vi "OP500InitParam.vi"(8 "errin":errorcluster, 11 "pathin":path) -> (0 "errout":errorcluster caption="error out")   [LabVIEW 2020]
uses:
  VG/VG_ISOmin.vi
  ZEN8 Semi Auto EMC/OP700/VG/VG_TCellmin.vi
  ZEN8 Semi Auto EMC/OP700/VG/VG_TCellmax.vi
  VG/VG_TusineMin.vi
  VG/VG_TusineMax.vi
  VG/VG_VCellMin30.vi
  VG/VG_VCellMax30.vi
  VG/VG_VCellMin70.vi
  VG/VG_VCellMax70.vi
  VG/VG_DeltaTcell.vi
  VG/VG_DeltaVcell.vi
  VG/VG_DCIRmin.vi
  VG/VG_DCIRmax.vi
  VG/VG_OCV30max.vi
  VG/VG_OCV30min.vi
  VG/VG_OCV70max.vi
  VG/VG_OCV70min.vi
  VG/VG_DCIRCurrent.vi
  VG/VG_EquipementsNeeded.vi
  VG/VG_DCIR+OUIouNON.vi
  VG/VG_OP400.vi
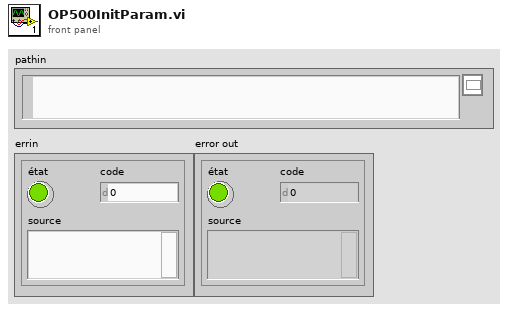
[diagram p1: front panel]
types:
  T1 = cluster{"[0]":dbl, "[1]":dbl, "[2]":dbl, "[3]":dbl, "[4]":dbl, "[5]":dbl, "[6]":dbl, "[7]":dbl, "[8]":dbl}
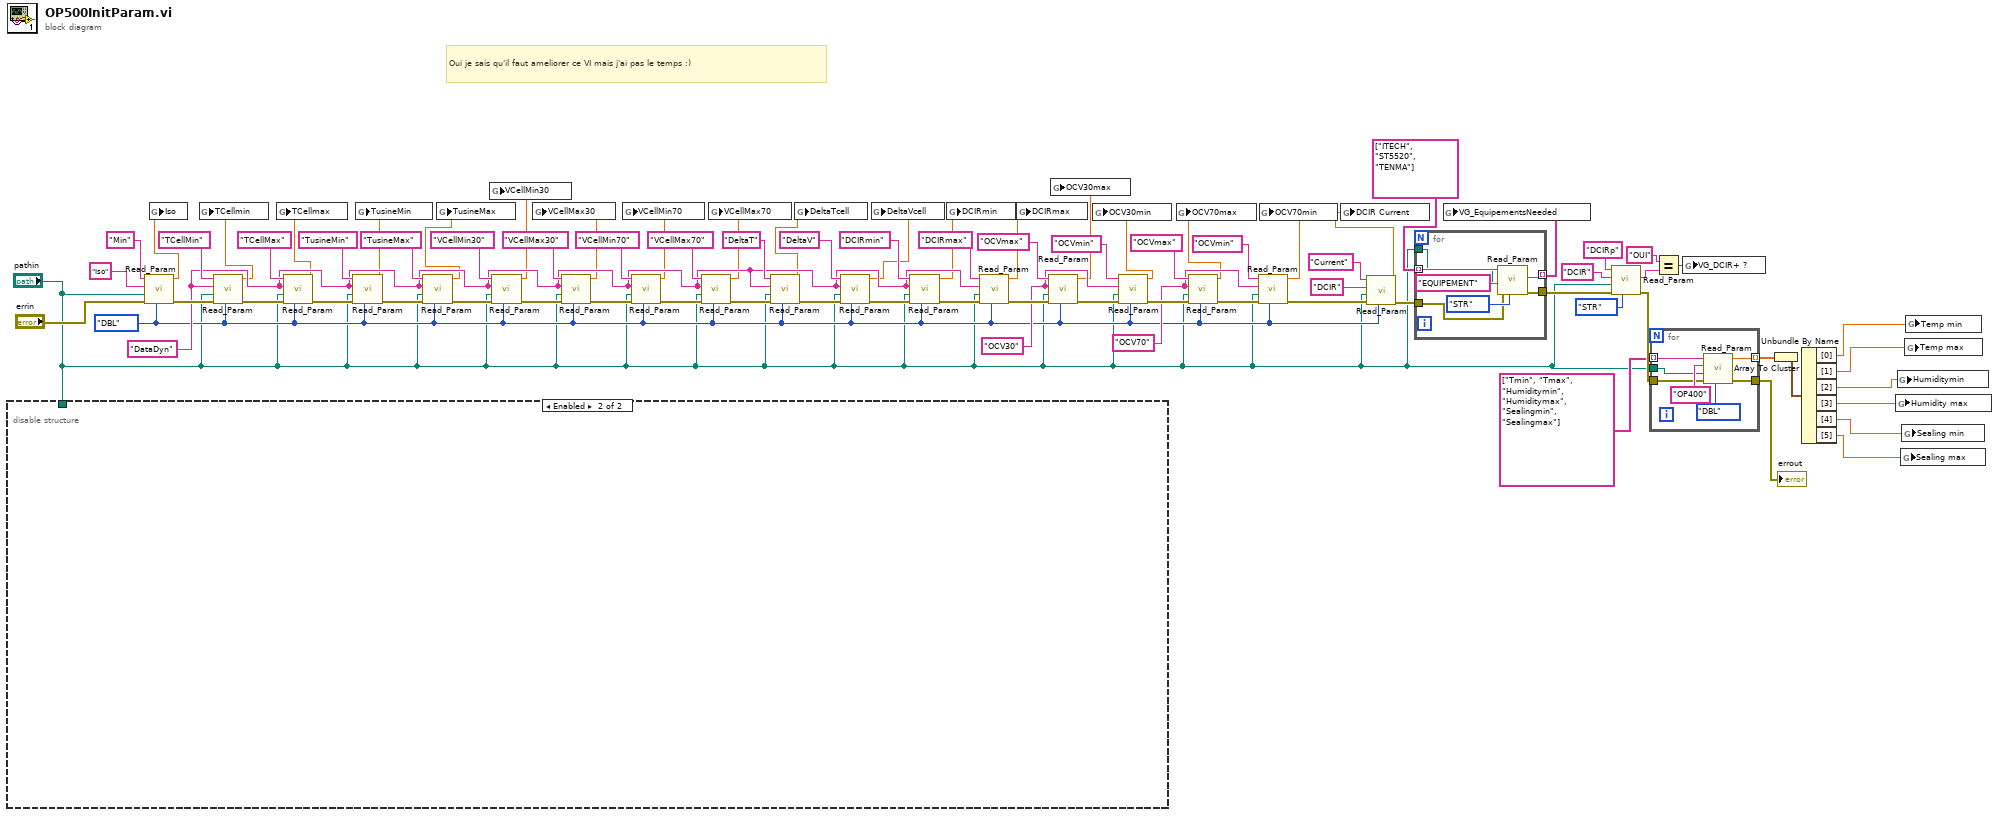
[diagram p0: block diagram]
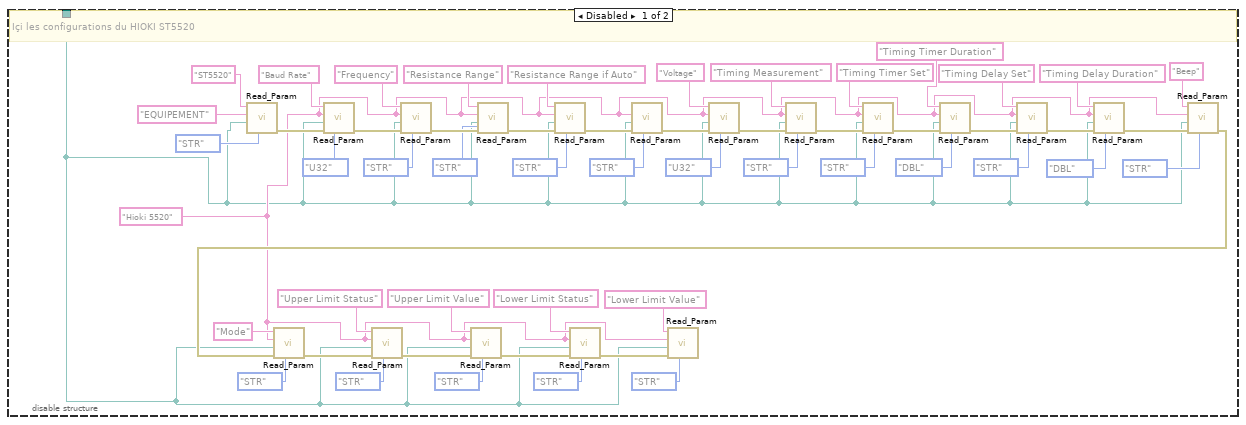
[diagram p2: hidden frame]
diagram:
  w45 = "OCV70" ("section")
  w47 = "OCV30" ("section")
  w51 = "DataDyn" ("section")
  w27 = enum16{"STR", "DBL", "U32", "chemin"}."DBL" ("Énum")
  # "Oui je sais qu'il faut ameliorer ce VI mais j'ai pas le temps :)"
  n1 = disable-structure shown="Enabled" {
    disable-tunnel: "pathin" -> [w83 _]
    frame Disabled {
      w85 = "Hioki 5520" ("section")
      # "Içi les configurations du HIOKI ST5520"
      n2 = call <userlib>:"Read_Param.vi"("Énum"=enum16{"STR", "DBL", "U32", "chemin"}."STR", "pathin"=w83, "section"="EQUIPEMENT", "key"="ST5520") -> ("error out"=w137:errorcluster)  [unwired: 3 in, 4 out]
      n3 = call <userlib>:"Read_Param.vi"("Énum"=enum16{"STR", "DBL", "U32", "chemin"}."U32", "errin"=w137, "pathin"=w83, "section"=w85, "key"="Baud Rate") -> ("error out"=w136:errorcluster)  [unwired: 2 in, 4 out]
      n4 = call <userlib>:"Read_Param.vi"("Énum"=enum16{"STR", "DBL", "U32", "chemin"}."STR", "errin"=w136, "pathin"=w83, "section"=w85, "key"="Frequency") -> ("error out"=w135:errorcluster)  [unwired: 2 in, 4 out]
      n5 = call <userlib>:"Read_Param.vi"("Énum"=enum16{"STR", "DBL", "U32", "chemin"}."STR", "errin"=w135, "pathin"=w83, "section"=w85, "key"="Resistance Range") -> ("error out"=w134:errorcluster)  [unwired: 2 in, 4 out]
      n6 = call <userlib>:"Read_Param.vi"("Énum"=enum16{"STR", "DBL", "U32", "chemin"}."STR", "errin"=w134, "pathin"=w83, "section"=w85, "key"="Resistance Range if Auto") -> ("error out"=w133:errorcluster)  [unwired: 2 in, 4 out]
      n7 = call <userlib>:"Read_Param.vi"("Énum"=enum16{"STR", "DBL", "U32", "chemin"}."STR", "errin"=w133, "pathin"=w83, "section"=w85) -> ("error out"=w132:errorcluster)  [unwired: 3 in, 4 out]
      n8 = call <userlib>:"Read_Param.vi"("Énum"=enum16{"STR", "DBL", "U32", "chemin"}."U32", "errin"=w132, "pathin"=w83, "section"=w85, "key"="Voltage") -> ("error out"=w131:errorcluster)  [unwired: 2 in, 4 out]
      n9 = call <userlib>:"Read_Param.vi"("Énum"=enum16{"STR", "DBL", "U32", "chemin"}."STR", "errin"=w131, "pathin"=w83, "section"=w85, "key"="Timing Measurement") -> ("error out"=w130:errorcluster)  [unwired: 2 in, 4 out]
      n10 = call <userlib>:"Read_Param.vi"("Énum"=enum16{"STR", "DBL", "U32", "chemin"}."STR", "errin"=w130, "pathin"=w83, "section"=w85, "key"="Timing Timer Set") -> ("error out"=w129:errorcluster)  [unwired: 2 in, 4 out]
      n11 = call <userlib>:"Read_Param.vi"("Énum"=enum16{"STR", "DBL", "U32", "chemin"}."DBL", "errin"=w129, "pathin"=w83, "section"=w85, "key"="Timing Timer Duration") -> ("error out"=w128:errorcluster)  [unwired: 2 in, 4 out]
      n12 = call <userlib>:"Read_Param.vi"("Énum"=enum16{"STR", "DBL", "U32", "chemin"}."STR", "errin"=w128, "pathin"=w83, "section"=w85, "key"="Timing Delay Set") -> ("error out"=w127:errorcluster)  [unwired: 2 in, 4 out]
      n13 = call <userlib>:"Read_Param.vi"("Énum"=enum16{"STR", "DBL", "U32", "chemin"}."DBL", "errin"=w127, "pathin"=w83, "section"=w85, "key"="Timing Delay Duration") -> ("error out"=w102:errorcluster)  [unwired: 2 in, 4 out]
      n14 = call <userlib>:"Read_Param.vi"("Énum"=enum16{"STR", "DBL", "U32", "chemin"}."STR", "errin"=w102, "pathin"=w83, "section"=w85, "key"="Beep") -> ("error out"=w100:errorcluster)  [unwired: 2 in, 4 out]
      n15 = call <userlib>:"Read_Param.vi"("Énum"=enum16{"STR", "DBL", "U32", "chemin"}."STR", "errin"=w100, "pathin"=w83, "section"=w85, "key"="Mode") -> ("error out"=w99:errorcluster)  [unwired: 2 in, 4 out]
      n16 = call <userlib>:"Read_Param.vi"("Énum"=enum16{"STR", "DBL", "U32", "chemin"}."STR", "errin"=w99, "pathin"=w83, "section"=w85, "key"="Upper Limit Status") -> ("error out"=w98:errorcluster)  [unwired: 2 in, 4 out]
      n17 = call <userlib>:"Read_Param.vi"("Énum"=enum16{"STR", "DBL", "U32", "chemin"}."STR", "errin"=w98, "pathin"=w83, "section"=w85, "key"="Upper Limit Value") -> ("error out"=w97:errorcluster)  [unwired: 2 in, 4 out]
      n18 = call <userlib>:"Read_Param.vi"("Énum"=enum16{"STR", "DBL", "U32", "chemin"}."STR", "errin"=w97, "pathin"=w83, "section"=w85, "key"="Lower Limit Status") -> ("error out"=w96:errorcluster)  [unwired: 2 in, 4 out]
      n19 = call <userlib>:"Read_Param.vi"("Énum"=enum16{"STR", "DBL", "U32", "chemin"}."STR", "errin"=w96, "pathin"=w83, "section"=w85, "key"="Lower Limit Value") -> ()  [unwired: 2 in, 5 out]
    }
    frame Enabled {
    }
  }
  n20 = call <userlib>:"Read_Param.vi"("Énum"=w27, "errin"="errin", "pathin"="pathin", "section"="Iso", "key"="Min") -> ("error out"=w79:errorcluster, "dbl"=w44:dbl)  [unwired: 2 in, 3 out]
  n21 = global write "VG_ISOmin.vi" "Iso"(w44) -> ()
  n22 = call <userlib>:"Read_Param.vi"("Énum"=w27, "errin"=w79, "pathin"="pathin", "section"=w51, "key"="TCellMin") -> ("error out"=w78:errorcluster, "dbl"=w43:dbl)  [unwired: 2 in, 3 out]
  n23 = global write "VG_TCellmin.vi" "TCellmin"(w43) -> ()
  n24 = call <userlib>:"Read_Param.vi"("Énum"=w27, "errin"=w78, "pathin"="pathin", "section"=w51, "key"="TCellMax") -> ("error out"=w77:errorcluster, "dbl"=w42:dbl)  [unwired: 2 in, 3 out]
  n25 = global write "VG_TCellmax.vi" "TCellmax"(w42) -> ()
  n26 = call <userlib>:"Read_Param.vi"("Énum"=w27, "errin"=w77, "pathin"="pathin", "section"=w51, "key"="TusineMin") -> ("error out"=w76:errorcluster, "dbl"=w41:dbl)  [unwired: 2 in, 3 out]
  n27 = global write "VG_TusineMin.vi" "TusineMin"(w41) -> ()
  n28 = call <userlib>:"Read_Param.vi"("Énum"=w27, "errin"=w76, "pathin"="pathin", "section"=w51, "key"="TusineMax") -> ("error out"=w75:errorcluster, "dbl"=w40:dbl)  [unwired: 2 in, 3 out]
  n29 = global write "VG_TusineMax.vi" "TusineMax"(w40) -> ()
  n30 = call <userlib>:"Read_Param.vi"("Énum"=w27, "errin"=w75, "pathin"="pathin", "section"=w51, "key"="VCellMin30") -> ("error out"=w74:errorcluster, "dbl"=w38:dbl)  [unwired: 2 in, 3 out]
  n31 = global write "VG_VCellMin30.vi" "VCellMin30"(w38) -> ()
  n32 = call <userlib>:"Read_Param.vi"("Énum"=w27, "errin"=w74, "pathin"="pathin", "section"=w51, "key"="VCellMax30") -> ("error out"=w73:errorcluster, "dbl"=w39:dbl)  [unwired: 2 in, 3 out]
  n33 = global write "VG_VCellMax30.vi" "VCellMax30"(w39) -> ()
  n34 = call <userlib>:"Read_Param.vi"("Énum"=w27, "errin"=w73, "pathin"="pathin", "section"=w51, "key"="VCellMin70") -> ("error out"=w72:errorcluster, "dbl"=w37:dbl)  [unwired: 2 in, 3 out]
  n35 = global write "VG_VCellMin70.vi" "VCellMin70"(w37) -> ()
  n36 = call <userlib>:"Read_Param.vi"("Énum"=w27, "errin"=w72, "pathin"="pathin", "section"=w51, "key"="VCellMax70") -> ("error out"=w71:errorcluster, "dbl"=w36:dbl)  [unwired: 2 in, 3 out]
  n37 = global write "VG_VCellMax70.vi" "VCellMax70"(w36) -> ()
  n38 = call <userlib>:"Read_Param.vi"("Énum"=w27, "errin"=w71, "pathin"="pathin", "section"=w51, "key"="DeltaT") -> ("error out"=w70:errorcluster, "dbl"=w35:dbl)  [unwired: 2 in, 3 out]
  n39 = global write "VG_DeltaTcell.vi" "DeltaTcell"(w35) -> ()
  n40 = call <userlib>:"Read_Param.vi"("Énum"=w27, "errin"=w70, "pathin"="pathin", "section"=w51, "key"="DeltaV") -> ("error out"=w69:errorcluster, "dbl"=w20:dbl)  [unwired: 2 in, 3 out]
  n41 = global write "VG_DeltaVcell.vi" "DeltaVcell"(w20) -> ()
  n42 = call <userlib>:"Read_Param.vi"("Énum"=w27, "errin"=w69, "pathin"="pathin", "section"=w51, "key"="DCIRmin") -> ("error out"=w68:errorcluster, "dbl"=w34:dbl)  [unwired: 2 in, 3 out]
  n43 = global write "VG_DCIRmin.vi" "DCIRmin"(w34) -> ()
  n44 = call <userlib>:"Read_Param.vi"("Énum"=w27, "errin"=w68, "pathin"="pathin", "section"=w51, "key"="DCIRmax") -> ("error out"=w67:errorcluster, "dbl"=w33:dbl)  [unwired: 2 in, 3 out]
  n45 = global write "VG_DCIRmax.vi" "DCIRmax"(w33) -> ()
  n46 = call <userlib>:"Read_Param.vi"("Énum"=w27, "errin"=w67, "pathin"="pathin", "section"=w47, "key"="OCVmax") -> ("error out"=w66:errorcluster, "dbl"=w32:dbl)  [unwired: 2 in, 3 out]
  n47 = global write "VG_OCV30max.vi" "OCV30max"(w32) -> ()
  n48 = call <userlib>:"Read_Param.vi"("Énum"=w27, "errin"=w66, "pathin"="pathin", "section"=w47, "key"="OCVmin") -> ("error out"=w65:errorcluster, "dbl"=w31:dbl)  [unwired: 2 in, 3 out]
  n49 = global write "VG_OCV30min.vi" "OCV30min"(w31) -> ()
  n50 = call <userlib>:"Read_Param.vi"("Énum"=w27, "errin"=w65, "pathin"="pathin", "section"=w45, "key"="OCVmax") -> ("error out"=w64:errorcluster, "dbl"=w30:dbl)  [unwired: 2 in, 3 out]
  n51 = global write "VG_OCV70max.vi" "OCV70max"(w30) -> ()
  n52 = call <userlib>:"Read_Param.vi"("Énum"=w27, "errin"=w64, "pathin"="pathin", "section"=w45, "key"="OCVmin") -> ("error out"=w28:errorcluster, "dbl"=w29:dbl)  [unwired: 2 in, 3 out]
  n53 = global write "VG_OCV70min.vi" "OCV70min"(w29) -> ()
  n54 = call <userlib>:"Read_Param.vi"("Énum"=w27, "errin"=w28, "pathin"="pathin", "section"="DCIR", "key"="Current") -> ("error out"=w22:errorcluster, "dbl"=w24:dbl)  [unwired: 2 in, 3 out]
  n55 = global write "VG_DCIRCurrent.vi" "DCIR Current"(w24) -> ()
  n56 = for {
    tunnel: string[] ["ITECH", "ST5520", "TENMA"] -> [w144] mode=indexing
    tunnel: w22 -> [w141]
    tunnel: [w138] -> w19
    tunnel: [w140] -> w21 mode=indexing
    tunnel: "pathin" -> [w139]
    n57 = call <userlib>:"Read_Param.vi"("Énum"=enum16{"STR", "DBL", "U32", "chemin"}."STR", "errin"=w141, "pathin"=w139, "section"="EQUIPEMENT", "key"=w144) -> ("error out"=w138:errorcluster, "str"=w140:string)  [unwired: 2 in, 3 out]
  }
  n58 = global write "VG_EquipementsNeeded.vi" "VG_EquipementsNeeded"(w21) -> ()
  n59 = call <userlib>:"Read_Param.vi"("Énum"=enum16{"STR", "DBL", "U32", "chemin"}."STR", "errin"=w19, "pathin"="pathin", "section"="DCIR", "key"="DCIRp") -> ("error out"=w12:errorcluster, "str"=w15:string)  [unwired: 2 in, 3 out]
  n60 = for {
    tunnel: w12 -> [w150]
    tunnel: [w149] -> w11
    tunnel: string[] ["Tmin", "Tmax", "Humiditymin", "Humiditymax", "Sealingmin", "Sealingmax"] -> [w148] mode=indexing
    tunnel: "pathin" -> [w146]
    tunnel: [w145] -> w8 mode=indexing
    n61 = call <userlib>:"Read_Param.vi"("Énum"=enum16{"STR", "DBL", "U32", "chemin"}."DBL", "errin"=w150, "pathin"=w146, "section"="OP400", "key"=w148) -> ("error out"=w149:errorcluster, "dbl"=w145:dbl)  [unwired: 2 in, 3 out]
  }
  "errout" <- w11
  n62 = Equal?(x="OUI" ("key"), y=w15) -> (x = y?=w13:bool)
  n63 = global write "VG_DCIR+OUIouNON.vi" "VG_DCIR+ ?"(w13) -> ()
  n64 = Array To Cluster(array=w8) -> (cluster=w7:T1)
  n65 = Unbundle By Name(w7) -> ("[0]"=w6:dbl, "[1]"=w5:dbl, "[2]"=w4:dbl, "[3]"=w3:dbl, "[4]"=w2:dbl, "[5]"=w1:dbl)
  n66 = global write "VG_OP400.vi" "Humidity max"(w3) -> ()
  n67 = global write "VG_OP400.vi" "Humiditymin"(w4) -> ()
  n68 = global write "VG_OP400.vi" "Sealing max"(w1) -> ()
  n69 = global write "VG_OP400.vi" "Sealing min"(w2) -> ()
  n70 = global write "VG_OP400.vi" "Temp max"(w5) -> ()
  n71 = global write "VG_OP400.vi" "Temp min"(w6) -> ()
